vi "Suite from Project.vi"(8 "error in (no error)":errorcluster, 10 "Project Path":path, 11 "LUnit Test Suite In":refnum<class "LUnit Test Suite.lvclass">) -> (0 "error out":errorcluster, 3 "LUnit Test Suite Out":refnum<class "LUnit Test Suite.lvclass">)   [LabVIEW 2020, in "Test Suite Factory.lvclass"]
doc: "Produce a test suite including all tests in a .lvproj file. This works recursively for nested projects."
uses:
  Test Suite Factory.lvclass
  LUnit Test Suite/LUnit Test Suite.lvclass
  C:/git/astemes-lunit/source/Core/Runnable/Runnable.lvclass
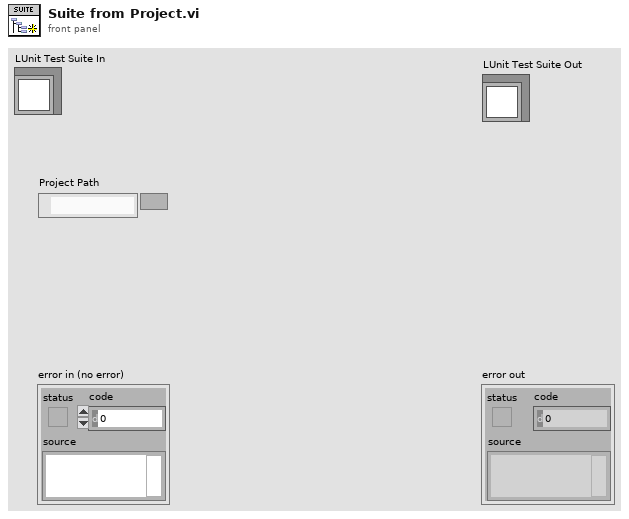
[diagram p1: front panel]
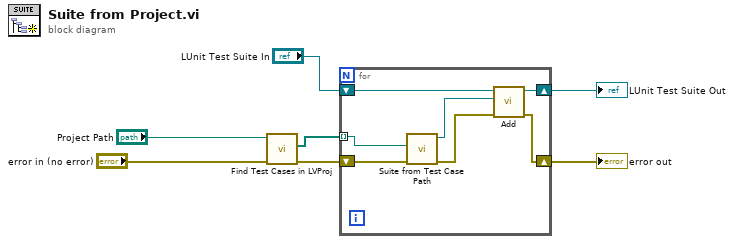
[diagram p0: block diagram]
diagram:
  n1 = call "Find Test Cases in LVProj.vi"("error in (no error)"="error in (no error)", "Project Path"="Project Path") -> ("error out"=w5:errorcluster, "Test Class paths"=w6:path[])  [unwired: 8 in]
  n2 = for {
    tunnel: w6 -> [w11] mode=indexing
    shift-right: [w13] -> w1
    shift-left: "LUnit Test Suite In" -> [w14]
    shift-right: [w12] -> w3
    shift-left: w5 -> [w8]
    n3 = call "Suite from Test Case Path.vi"("error in (no error)"=w8, "Test Case"=w11) -> ("error out"=w10:errorcluster, "LUnit Test Suite Out"=w9:refnum<class "LUnit Test Suite.lvclass">)  [unwired: 8 in]
    n4 = call "Add.vi"("error in (no error)"=w10, "Runnable"=w9, "LUnit Test Suite In"=w14) -> ("error out"=w12:errorcluster, "LUnit Test Suite Out"=w13:refnum<class "LUnit Test Suite.lvclass">)  [unwired: 7 in]
  }
  "error out" <- w3
  "LUnit Test Suite Out" <- w1
